vi "distancepidinit.vi"() -> ()   [LabVIEW 2013]
uses:
  <vilib>/addons/control/pid/NI_PID_pid.lvlib
  <vilib>/addons/control/pid/pid.llb/PID (DBL).vi
panel:
  in  "reinitialize? (F)":bool
  out "Done?":bool
  in  "Adjustment Variable":dbl=0.72
  in  "PID Gains Distance":T1={"proportional gain (Kc)"=1.0, "integral time (Ti, min)"=0.01, "derivative time (Td, min)"=0.0} {"derivative time (Td, min)" format="%.3f"; "integral time (Ti, min)" format="%.3f"; "proportional gain (Kc)" format="%.3f"}
  in  "Distance From Target":dbl
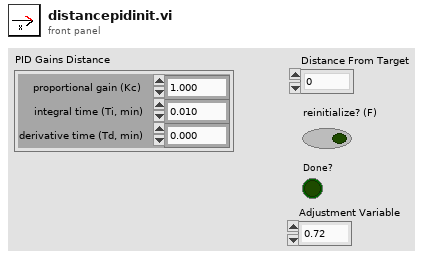
[diagram p1: front panel]
types:
  T1 = cluster{"proportional gain (Kc)":dbl, "integral time (Ti, min)":dbl, "derivative time (Td, min)":dbl}
  T2 = typedef "WPI_EncoderDevRef.ctl" = cluster{"DevStatus":errorcluster, "EncoderIndex":T3, "CounterIndex":T4, "DistancePerCount":dbl, "Decoding Type":T5}
  T3 = typedef "FPGA_EncoderIdx.ctl" = enum8{"Enc 0", "Enc 1", "Enc 2", "Enc 3", "Invalid"}
  T4 = typedef "FPGA_CounterCtrSystemIndex.ctl" = enum8{"Ctr 0", "Ctr 1", "Ctr 2", "Ctr 3", "Ctr 4", "Ctr 5", "Ctr 6", "Ctr 7", "Invalid"}
  T5 = typedef "WPI_EncoderType.ctl" = enum16{"1x", "2x", "4x"}
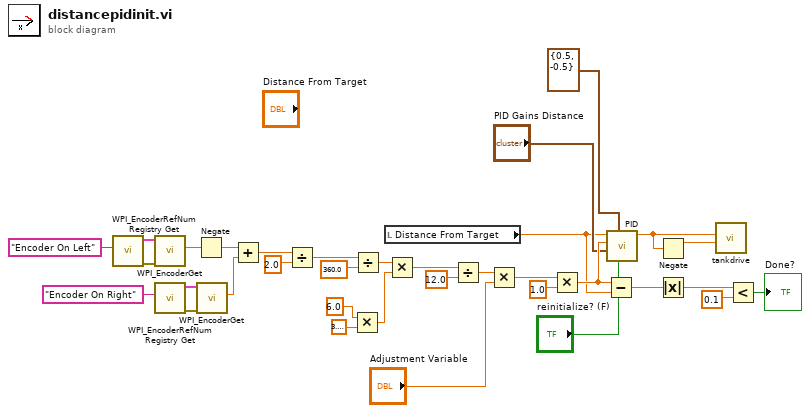
[diagram p0: block diagram]
diagram:
  n1 = call <vilib>:"WPI_EncoderRefNum Registry Get.vi"("refnum name"="Encoder On Left") -> ("error out"=w15:errorcluster, "EncoderDevRef"=w16:T2)  [unwired: 9 in]
  n2 = call <vilib>:"WPI_EncoderGet.vi"("error in (no error)"=w15, "EncoderDevRef"=w16) -> ("Distance"=w10:dbl)  [unwired: 4 in, 5 out]
  n3 = call <vilib>:"WPI_EncoderRefNum Registry Get.vi"("refnum name"="Encoder On Right") -> ("error out"=w17:errorcluster, "EncoderDevRef"=w18:T2)  [unwired: 9 in]
  n4 = Negate(x=w10) -> (-x=w9:dbl)
  n5 = call <vilib>:"WPI_EncoderGet.vi"("error in (no error)"=w17, "EncoderDevRef"=w18) -> ("Distance"=w21:dbl)  [unwired: 4 in, 5 out]
  n6 = Add(x=w9, y=w21) -> (x+y=w22:dbl)
  n7 = Divide(x=w22, y=2.0) -> (x/y=w26:dbl)
  n8 = Multiply(x=6.0, y=3.141592653589793) -> (x*y=w29:dbl)
  n9 = Divide(x=w26, y=360.0) -> (x/y=w28:dbl)
  n10 = local read "Distance From Target"() -> (w4:dbl)
  n11 = Multiply(x=w28, y=w29) -> (x*y=w30:dbl)
  n12 = Divide(x=w30, y=12.0) -> (x/y=w13:dbl)
  n13 = Multiply(x=w13, y="Adjustment Variable") -> (x*y=w12:dbl)
  n14 = Multiply(x=w12, y=1.0) -> (x*y=w8:dbl)
  n15 = Subtract(x=w8, y=w4) -> (x-y=w32:dbl)
  n16 = call-poly <vilib>:"PID.vi"("reinitialize? (F)"="reinitialize? (F)", "output range"=cluster{"output high":dbl, "output low":dbl} {"output high"=0.5, "output low"=-0.5}, "PID gains"="PID Gains Distance", "process variable"=w8, "setpoint"=w4) -> ("output"=w2:dbl)  [unwired: 5 in, 1 out]
  n17 = Negate(x=w2) -> (-x=w1:dbl)
  n18 = Absolute Value(x=w32) -> (abs(x)=w33:dbl)
  n19 = call "tankdrive.vi"("Right Value"=w1, "Left Value"=w2) -> ()  [unwired: 10 in]
  n20 = Less?(x=w33, y=0.1) -> (x < y?=→"Done?":bool)
